vi "Delete.vi"(6 "TableName":string, 7 "condition":string, 8 "error in (no error)":errorcluster, 11 "DataBase_SQL in":refnum<class "DataBase_SQL.lvclass">) -> (0 "error out":errorcluster, 3 "DataBase_SQL out":refnum<class "DataBase_SQL.lvclass">)   [LabVIEW 2021, in "DataBase_SQL.lvclass"]
uses:
  <userlib>/John_Lib/DataBase/DataBase_SQL/DataBase_SQL.lvclass
  <userlib>/John_Lib/DataBase/DataBase_SQL/DataBase_SQL.lvclass/DataBase_SQL.ctl
panel:
  out "SQL Query":string
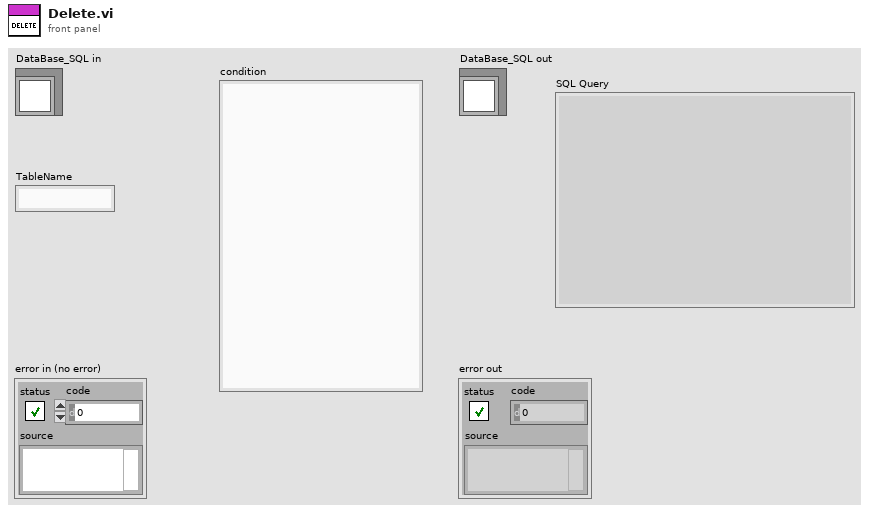
[diagram p1: front panel]
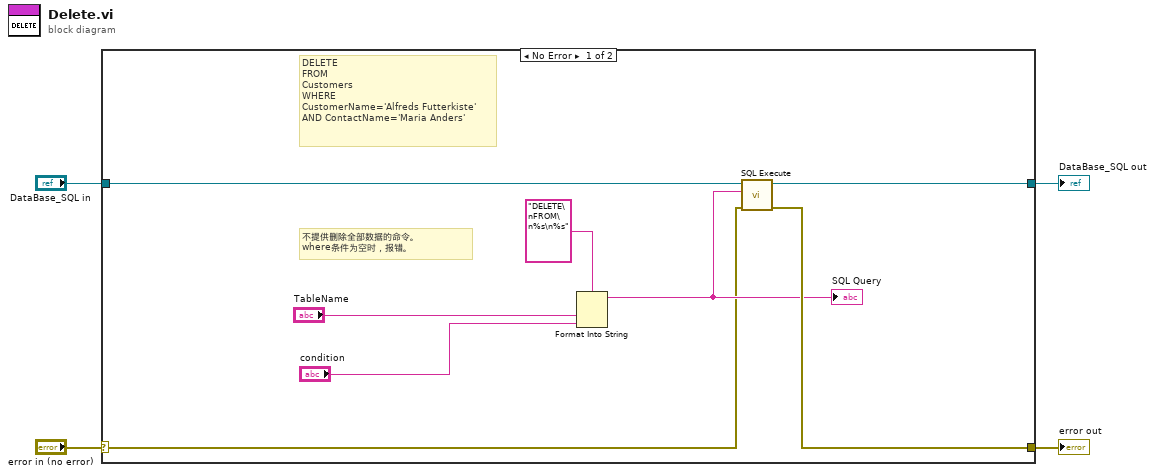
[diagram p0: block diagram]
diagram:
  n1 = case shown="No Error" "error in (no error)" {
    selector: "error in (no error)" -> [w6 w14]
    tunnel: [w9 w14] -> w3
    tunnel: [w7 w13] -> w1
    tunnel: "DataBase_SQL in" -> [w10 w13]
    frame No Error {
      # "不提供删除全部数据的命令。\nwhere条件为空时，报错。"
      # "DELETE\nFROM\nCustomers\nWHERE\nCustomerName='Alfreds Futterkiste'\nAND ContactName='Maria Anders'"
      n2 = Format Into String(format string="DELETE\nFROM\n%s\n%s", "TableName", "condition") -> (resulting string=w8:string)  [unwired: 2 in, 1 out]
      "SQL Query" <- w8
      n3 = call-dynamic "SQL Execute.vi"("error in (no error)"=w6, "Command Text"=w8, "DataBase_SQL in"=w10) -> ("error out"=w9:errorcluster, "DataBase_SQL out"=w7:refnum<class "DataBase_SQL.lvclass">)  [unwired: 4 in, 3 out]
    }
    frame Error {
    }
  }
  "error out" <- w3
  "DataBase_SQL out" <- w1
